vi "In Use.vi"(0 "SignalManager in":refnum<class "SignalManager.lvclass">, 11 "error in (no error)":errorcluster) -> (4 "SignalManager out":refnum<class "SignalManager.lvclass">, 8 "In use":bool, 15 "error out":errorcluster)   [LabVIEW 2015, in "SignalManager.lvclass"]
uses:
  SignalManager.lvclass
  SignalManager.lvclass/SignalManager.ctl
  Channel/Channel.lvclass/Channel.ctl
  Channel/Read Waveform.vi
  Waveforms/Waveform/Waveform.lvclass
  Koop/KObject Class/KObject.lvclass
  Channel/Channel.lvclass
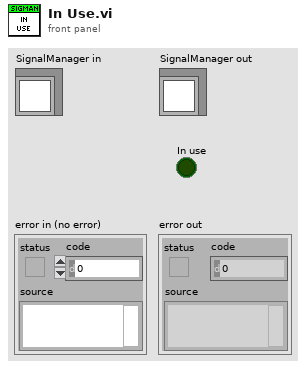
[diagram p1: front panel]
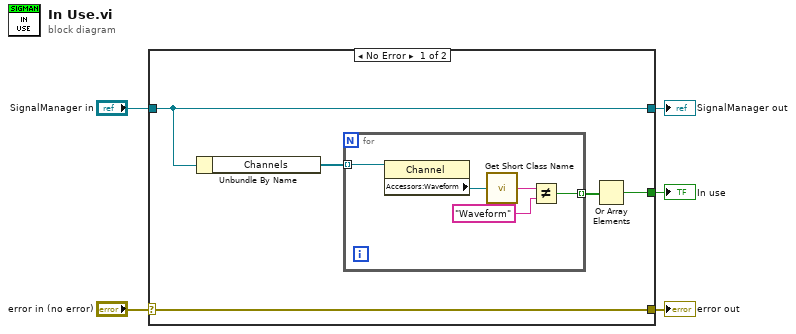
[diagram p0: block diagram]
diagram:
  n1 = case shown="No Error" "error in (no error)" {
    selector: "error in (no error)" -> [w10 w17]
    tunnel: [w10 w17] -> w4
    tunnel: [w9 w16] -> w2
    tunnel: "SignalManager in" -> [w9 w16]
    tunnel: [w6 _] -> w1
    frame No Error {
      n2 = Unbundle By Name(w9) -> ("Channels"=w8:refnum<class "Channel.lvclass">[])
      n3 = for {
        tunnel: w8 -> [w15] mode=indexing
        tunnel: [w11] -> w7 mode=indexing
        n4 = property class="Channel"(reference=w15) -> ("Accessors:Waveform"=w14:refnum<class "Waveform.lvclass">)  [unwired: 1 in, 2 out]
        n5 = call "Get Short Class Name.vi"("KObject in"=w14) -> ("Class"=w13:string)  [unwired: 4 in]
        n6 = Not Equal?(x=w13, y="Waveform") -> (x != y?=w11:bool)
      }
      n7 = Or Array Elements(Boolean array=w7) -> (logical OR=w6:bool)
    }
    frame Error {
    }
  }
  "error out" <- w4
  "SignalManager out" <- w2
  "In use" <- w1
